vi "createNewDocument.vi"(8 "error in (no error)":errorcluster, 10 "Document Path":path, 11 "workbook in":refnum<class "workbook.lvclass">) -> (0 "error out":errorcluster, 3 "workbook out":refnum<class "workbook.lvclass">)   [LabVIEW 2017, in "Excel_Specific.lvlib" / "workbook.lvclass"]
uses:
  workbook.lvclass
  C:/Users/Neo/Desktop/Dev_Tools_BR/LabVIEW_NPOI/src/LabVIEW NPOI/NPOI_Document/npoiDocument/npoiDocument.lvclass
  NPOI_Document/npoiDocument/npoiDocument.lvclass/npoiDocument.ctl
  xssfWorkbook/xssfWorkbook.lvclass
  C:/Users/Neo/Desktop/Dev_Tools_BR/LabVIEW_NPOI/src/LabVIEW NPOI/Excel_Specific/workbook/workbook.lvclass
  hssfWorkbook/hssfWorkbook.lvclass
  NPOI_Document/npoiDocument/Get Document.Path.vi
  NPOI_Document/npoiDocument/npoiDocument.lvclass
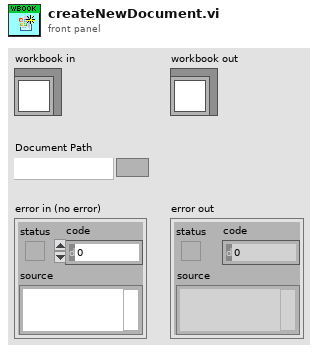
[diagram p1: front panel]
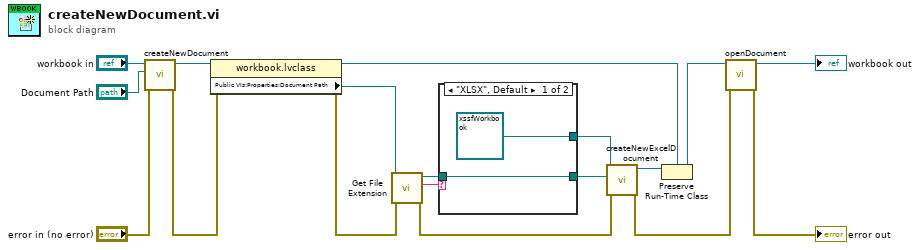
[diagram p0: block diagram]
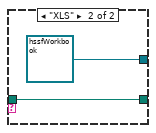
[diagram p2: hidden frame]
diagram:
  n1 = call-parent "createNewDocument.vi"("error in (no error)"="error in (no error)", "Document Path"="Document Path", "npoiDocument in"="workbook in") -> ("error out"=w13:errorcluster, "npoiDocument out"=w16:refnum<class "workbook.lvclass">)  [unwired: 7 in]
  n2 = property class="workbook.lvclass"(reference=w16, error in=w13) -> (reference out=w10:refnum<class "workbook.lvclass">, error out=w6:errorcluster, "Public VIs:Properties:Document Path"=w9:path)
  n3 = call <vilib>:"Get File Extension.vi"("error in (no error)"=w6, "file"=w9) -> ("error out"=w5:errorcluster, "lowercase file extension"=w18:string, "dup file"=w8:path)  [unwired: 5 in, 2 out]
  n4 = case shown="\"XLSX\", Default" w18 {
    tunnel: [refnum<class "xssfWorkbook.lvclass"> refnum ("Excel_Specific.lvlib:xssfWorkbook.lvclass") refnum<class "hssfWorkbook.lvclass"> refnum ("Excel_Specific.lvlib:hssfWorkbook.lvclass")] -> w12
    tunnel: w8 -> [w19 w21]
    tunnel: [w19 w21] -> w7
    frame "XLSX", Default {
    }
    frame "XLS" {
    }
  }
  n5 = call-dynamic "createNewExcelDocument.vi"("error in (no error)"=w5, "Excel File Path"=w7, "workbook in"=w12) -> ("error out"=w2:errorcluster, "workbook out"=w11:refnum<class "workbook.lvclass">)  [unwired: 7 in]
  n6 = Preserve Run-Time Class(object in=w11, 2:w10) -> (object out=w4:refnum<class "workbook.lvclass">)  [unwired: 1 in, 1 out]
  n7 = call-dynamic "openDocument.vi"("error in (no error)"=w2, "workbook in"=w4) -> ("error out"=→"error out":errorcluster, "workbook out"=→"workbook out":refnum<class "workbook.lvclass">)  [unwired: 8 in]
